vi "Get XY graph from TDMS file.vi"(8 "error in":errorcluster, 11 "TDMS file path":path) -> (0 "error out":errorcluster, 1 "graph":cluster{"X":dbl[], "Y":dbl[]}[](graph), 3 "TDMS file path out":path)   [LabVIEW 2025]
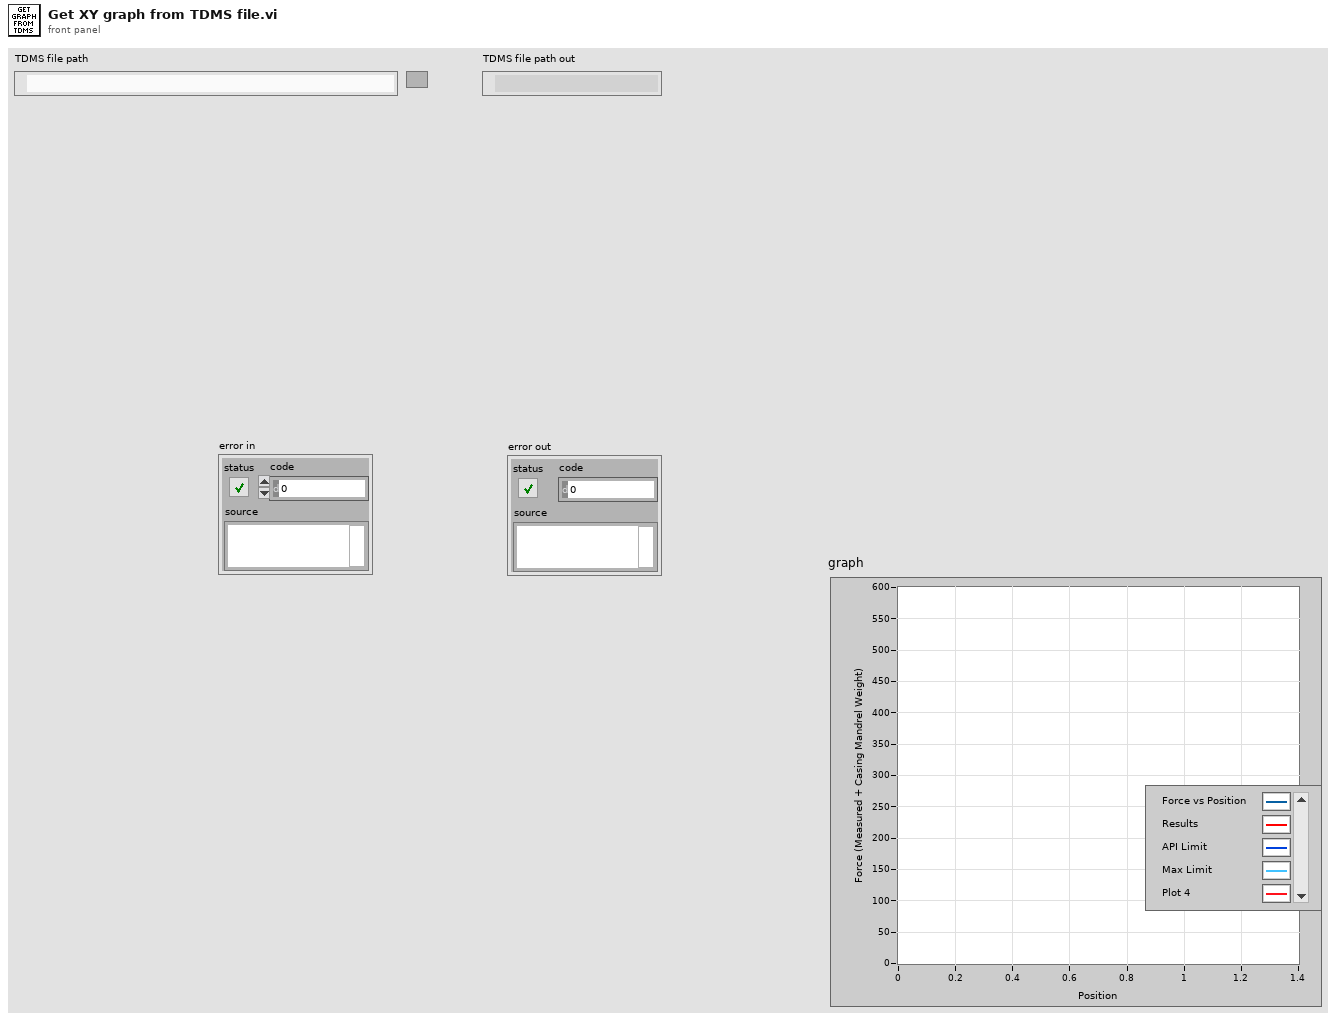
[diagram p1: front panel]
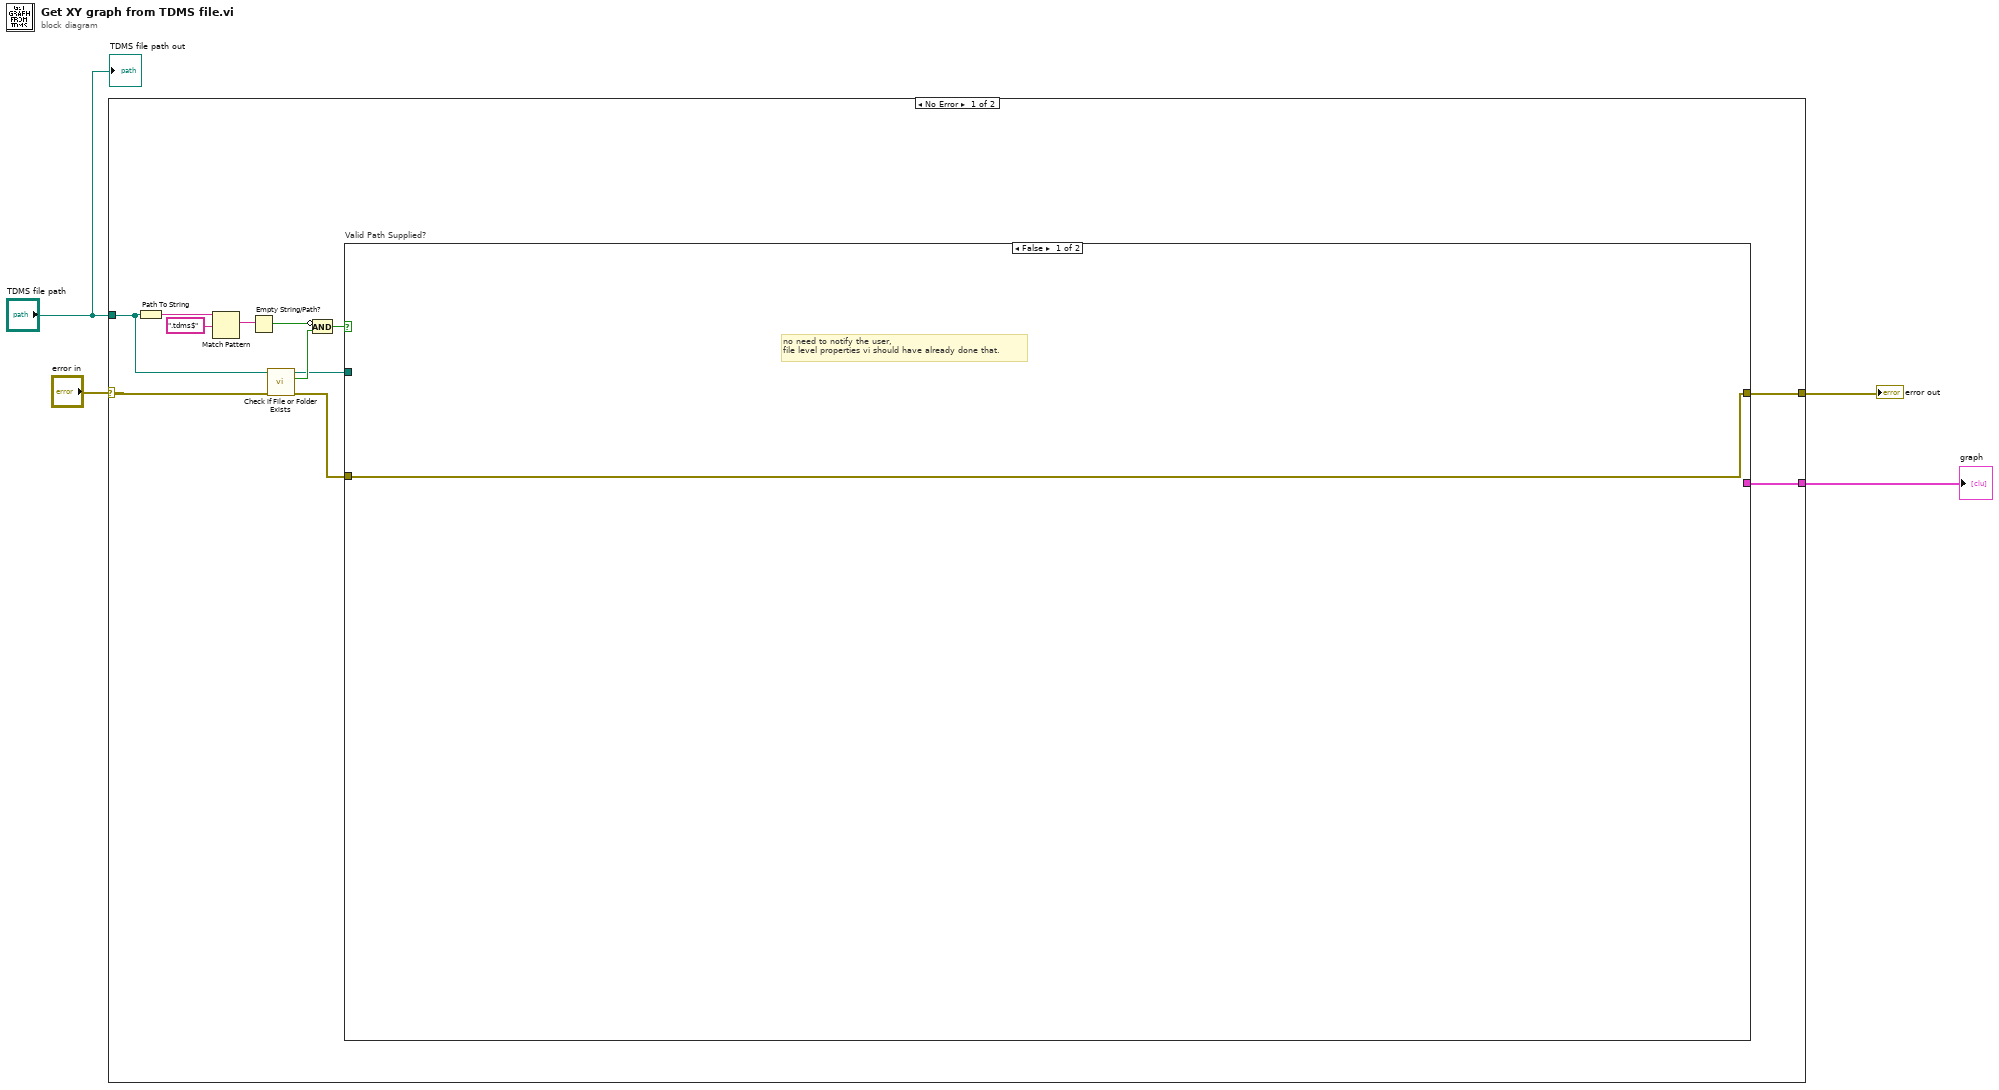
[diagram p0: block diagram]
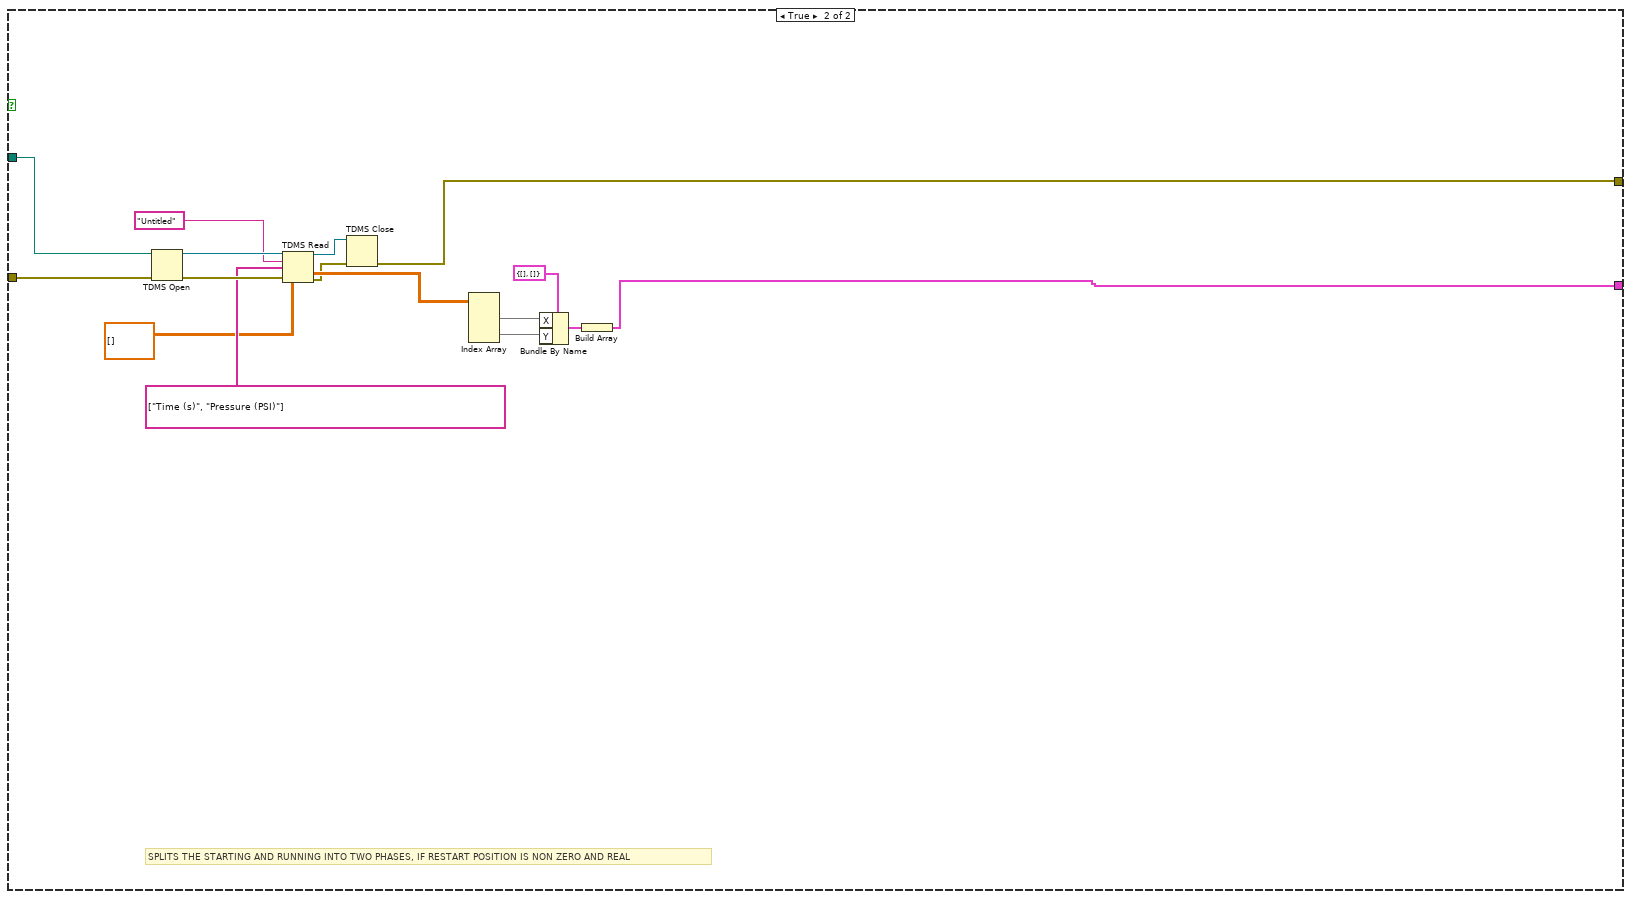
[diagram p2: hidden frame]
diagram:
  n1 = case shown="No Error" "error in" {
    selector: "error in" -> [w5 w34]
    tunnel: "TDMS file path" -> [w14 _]
    tunnel: [w9 w34] -> w2
    tunnel: [w8 _] -> w1
    frame No Error {
      n2 = Path To String(path=w14) -> (string=w15:string)
      n3 = Match Pattern(string=w15, regular expression=".tdms$") -> (match substring=w13:string)  [unwired: 1 in, 3 out]
      n4 = Empty String/Path?(string/path=w13) -> (empty?=w12:bool)
      n5 = call <vilib>:"Check if File or Folder Exists.vi"("error in (no error)"=w5, "path"=w14) -> ("error out"=w6:errorcluster, "file or folder exists?"=w11:bool, "dup path"=w7:path)  [unwired: 7 in]
      n6 = Compound Arithmetic op=AND(invert w12, w11) -> (w10:bool)
      n7 = case "Valid Path Supplied?" shown="False" w10 {
        tunnel: [w17 w18] -> w9
        tunnel: [_ w21] -> w8
        tunnel: w7 -> [_ w31]
        tunnel: w6 -> [w17 w30]
        frame False {
          # "no need to notify the user, \nfile level properties vi should have already done that."
        }
        frame True {
          # "SPLITS THE STARTING AND RUNNING INTO TWO PHASES, IF RESTART POSITION IS NON ZERO AND REAL"
          n8 = TDMS Open(8:w30, 11:w31) -> (0:w33:errorcluster, 3:w32:refnum<k34>)  [unwired: 5 in]
          n9 = TDMS Read(0:w32, 5:"Untitled" ("group name in"), 7:string[] ["Time (s)", "Pressure (PSI)"] ("channel name(s) in"), 11:w33, 12:dbl[][] [] ("Array")) -> (4:w20:refnum<k34>, 10:w25:dbl[][], 15:w19:errorcluster)  [unwired: 3 in, 3 out]
          n10 = TDMS Close(8:w19, 11:w20) -> (0:w18:errorcluster)  [unwired: 1 out]
          n11 = Index Array(array=w25) -> (element #1=w24:dbl[], element #2=w23:dbl[])  [unwired: 4 in]
          n12 = Bundle By Name(cluster=cluster{"X":dbl[], "Y":dbl[]} {"X"=[], "Y"=[]} ("Running Force Line"), "X"=w24, "Y"=w23) -> (w22:cluster{"X":dbl[], "Y":dbl[]})
          n13 = Build Array(w22) -> (w21:cluster{"X":dbl[], "Y":dbl[]}[])
        }
      }
    }
    frame Error {
    }
  }
  "error out" <- w2
  "graph" <- w1
  "TDMS file path out" <- "TDMS file path"
